vi "Get Connector Pane Type.vi"(7 "error in (no error)":errorcluster, 10 "Controls[]":refnum<vi>[](array[refnum])) -> (0 "error out":errorcluster, 2 "Connector Pane Type":T1)   [LabVIEW 2018, in "NISAST VI Scripting.lvlib" / "VI.lvlib" / "Connector.lvlib"]
uses:
  Connector/Connector.lvlib
  Attribute/Connector Pane Type.ctl
  Front Panel.lvlib
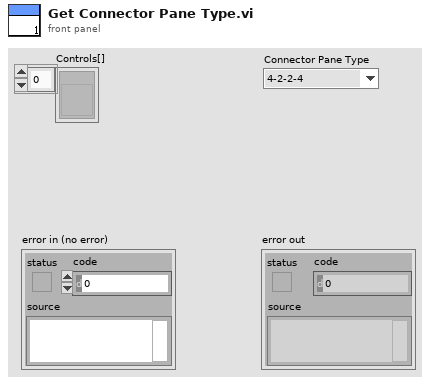
[diagram p1: front panel]
types:
  T1 = typedef "NISAST VI Scripting.lvlib/VI.lvlib/Front Panel.lvlib/Connector Pane Type.ctl" = enum16{"4-2-2-4", "5-2-2-2-5", "Others"}
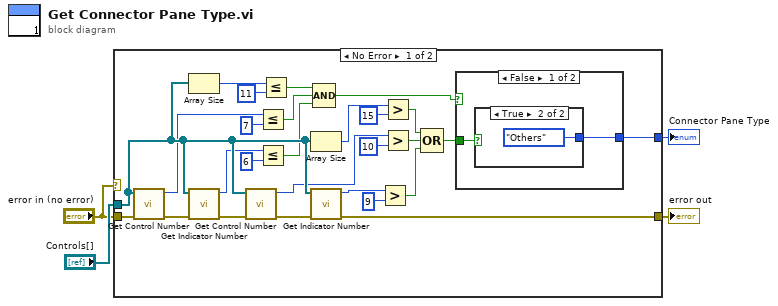
[diagram p0: block diagram]
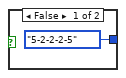
[diagram p2: hidden frame]
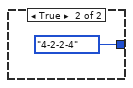
[diagram p3: hidden frame]
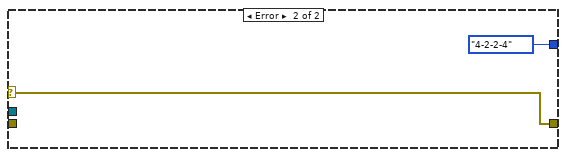
[diagram p4: hidden frame]
diagram:
  n1 = case shown="No Error" "error in (no error)" {
    selector: "error in (no error)" -> [_ w38]
    tunnel: "Controls[]" -> [w28 _]
    tunnel: [w10 Connector_Pane_Type."4-2-2-4" ("Connector Pane Type")] -> w3
    tunnel: "error in (no error)" -> [w9 _]
    tunnel: [w5 w38] -> w2
    frame No Error {
      n2 = call "Get Control Number.vi"("error in (no error)"=w9, "Controls[]"=w28) -> ("error out"=w8:errorcluster, "size(s)"=w15:i32)  [unwired: 1 in, 7 out]
      n3 = Array Size(array=w28) -> (size(s)=w13:i32)
      n4 = call "Get Indicator Number.vi"("error in (no error)"=w8, "Controls[]"=w28) -> ("error out"=w7:errorcluster, "size(s)"=w17:i32)  [unwired: 8 out]
      n5 = call "Get Control Number.vi"("error in (no error)"=w7, "Controls[]"=w28) -> ("error out"=w6:errorcluster, "size(s)"=w22:i32)  [unwired: 1 in, 7 out]
      n6 = Less Or Equal?(x=w15, y=7) -> (x <= y?=w20:bool)
      n7 = Less Or Equal?(x=w17, y=6) -> (x <= y?=w21:bool)
      n8 = Less Or Equal?(x=w13, y=11) -> (x <= y?=w19:bool)
      n9 = Array Size(array=w28) -> (size(s)=w26:i32)
      n10 = call "Get Indicator Number.vi"("error in (no error)"=w6, "Controls[]"=w28) -> ("error out"=w5:errorcluster, "size(s)"=w24:i32)  [unwired: 8 out]
      n11 = Compound Arithmetic op=AND(w19, w20, w21) -> (w12:bool)
      n12 = Greater?(x=w24, y=9) -> (0:w31:bool)
      n13 = Greater?(x=w26, y=15) -> (0:w29:bool)
      n14 = Greater?(x=w22, y=10) -> (0:w30:bool)
      n15 = Compound Arithmetic op=OR(w29, w30, w31) -> (w11:bool)
      n16 = case shown="False" w12 {
        tunnel: [w32 Connector_Pane_Type."4-2-2-4" ("Connector Pane Type")] -> w10
        tunnel: w11 -> [w33 _]
        frame False {
          n17 = case shown="True" w33 {
            tunnel: [Connector_Pane_Type."5-2-2-2-5" ("Connector Pane Type") Connector_Pane_Type."Others" ("Connector Pane Type")] -> w32
            frame False {
            }
            frame True {
            }
          }
        }
        frame True {
        }
      }
    }
    frame Error {
    }
  }
  "Connector Pane Type" <- w3
  "error out" <- w2
